vi "var_rx_stop.vi"() -> ()   [LabVIEW 2014]
panel:
  out "rx stop":bool
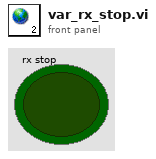
[diagram p1: front panel]
diagram:
